vi "Mode of Operation Value Change.vi"(8 "error in (no error)":errorcluster, 10 "Mode of Operation":T1, 11 "Doors Closing in":refnum<class "Doors Closing.lvclass">) -> (0 "error out":errorcluster, 3 "Doors Closing out":refnum<class "Doors Closing.lvclass">)   [LabVIEW 2020, in "Door Controller.lvlib" / "Doors Closing.lvclass"]
uses:
  Doors Closing.lvclass
  Door Interlocks/Mode of Operation.ctl
  Door Controller/Door Controller.lvclass
  Door Interlocks/Door Interlocks.lvclass
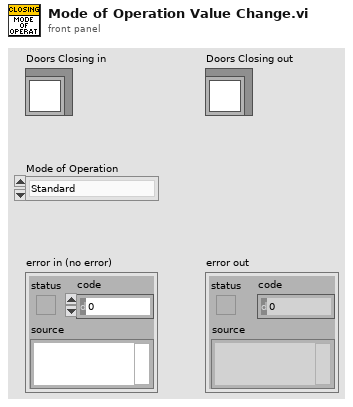
[diagram p1: front panel]
types:
  T1 = typedef "Door Interlocks.lvclass/Mode of Operation.ctl" = enum16{"Standard", "Interlock Override"}
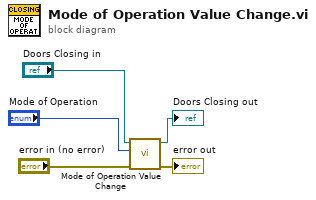
[diagram p0: block diagram]
diagram:
  n1 = call-parent "Mode of Operation Value Change.vi"("error in (no error)"="error in (no error)", "Mode of Operation"="Mode of Operation", "Door Controller in"="Doors Closing in") -> ("error out"=→"error out":errorcluster, "Door Controller out"=→"Doors Closing out":refnum<class "Doors Closing.lvclass">)  [unwired: 7 in]
